vi "pp2_updateSessionInfo.vi"(10 "Session info In":T1, 11 "State In":T2={"Curr  tr"=0, "Curr (ms)"=0, "Cum (ms)"=0, "Run loop diff"=0, "Tone countdown (ms)"=0, "Countdown (ms)"=0, "Curr State"=enum."0 NULL", "Prev State"=enum."0 NULL", "Null"=FALSE, "Sw"=FALSE, "Tone\nGate"=FALSE, "Stim"=FALSE, "Current DAQ DO Int"=0, "Current Loaded Trial"={"Trial Type Number"=1, "Trial Type"=enum."GO", "Trial Weight"=100, "Shock (mA)"=0.3, "Duration (ms)"=0.25, "Sound Type"=enum."04 FM Sweep", "Stim P1"=4000.0, "Stim P2"=0.0, "Stim P3"=0.0, "Stim P4"=2000.0}, "Next Trial (for display purposes)"={"Trial Type Number"=1, "Trial Type"=enum."GO", "Trial Weight"=100, "Shock (mA)"=0.3, "Duration (ms)"=0.25, "Sound Type"=enum."04 FM Sweep", "Stim P1"=4000.0, "Stim P2"=0.0, "Stim P3"=0.0, "Stim P4"=2000.0}, "Total trials memo"=0, "State start cum memo (ms)"=0, "Last dur jump time memo (ms)"=0, "Last dur shock time memo (ms)"=0, "Tone repeat memo (ms)"=0, "Webcam on"=FALSE, "Webcam recording"=FALSE, "State update flag"=FALSE, "Last loaded shock voltage"=0.0} {"Current DAQ DO Int" format="%016b"; "Next Trial (for display purposes)"."Shock (mA)" min=-1.0 max=5.0; "Next Trial (for display purposes)"."Trial Weight" step=1; "Next Trial (for display purposes)"."Duration (ms)" min=0.0 max=1.0; "Next Trial (for display purposes)"."Trial Type Number" min=1 step=1; "Current Loaded Trial"."Shock (mA)" min=-1.0 max=5.0; "Current Loaded Trial"."Trial Weight" step=1; "Current Loaded Trial"."Duration (ms)" min=0.0 max=1.0; "Current Loaded Trial"."Trial Type Number" min=1 step=1}) -> (2 "Session info Out":T1)   [LabVIEW 2013]
uses:
  pp2_CTL_StateInfo.ctl
  pp2_CTL_State.ctl
  pp2_Trial.ctl
  pp2_CTL_TrialType.ctl
  labolabo2/waveforms/WFTypes.ctl
  pp2_CTL_SessionInfo.ctl
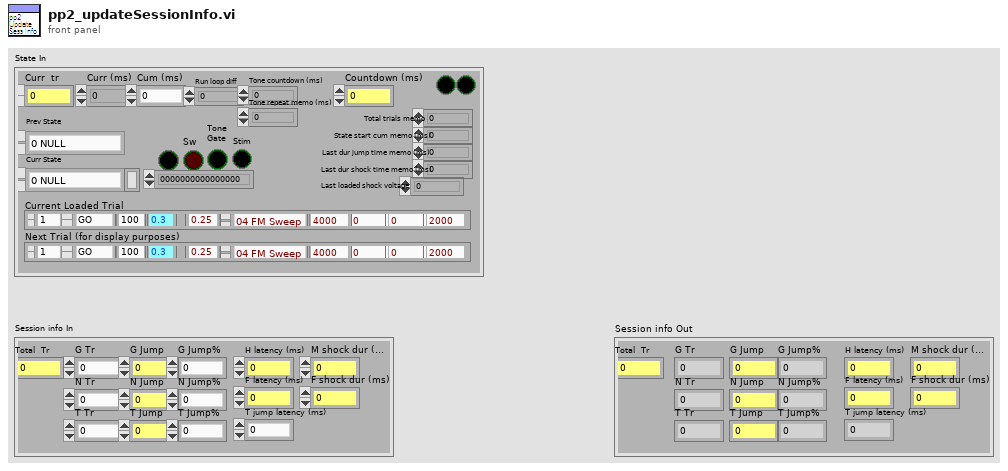
[diagram p1: front panel]
types:
  T1 = typedef "pp2_CTL_SessionInfo.ctl" = cluster{"Total  Tr":u32, "G Tr":u32, "G Jump":u32, "G Jump%":dbl, "N Tr":u32, "N Jump":u32, "N Jump%":dbl, "T Tr":u32, "T Jump":u32, "T Jump%":dbl, "M shock dur (ms)":dbl, "F shock dur (ms)":dbl, "H latency (ms)":dbl, "F latency (ms)":dbl, "T jump latency (ms)":dbl}
  T2 = typedef "pp2_CTL_StateInfo.ctl" = cluster{"Curr  tr":u16, "Curr (ms)":u32, "Cum (ms)":i64, "Run loop diff":i64, "Tone countdown (ms)":i64, "Countdown (ms)":i64, "Curr State":T3, "Prev State":T3, "Null":bool, "Sw":bool, "Tone\nGate":bool, "Stim":bool, "Current DAQ DO Int":u16, "Current Loaded Trial":T4, "Next Trial (for display purposes)":T4, "Total trials memo":i64, "State start cum memo (ms)":i64, "Last dur jump time memo (ms)":i64, "Last dur shock time memo (ms)":i64, "Tone repeat memo (ms)":i64, "Webcam on":bool, "Webcam recording":bool, "State update flag":bool, "Last loaded shock voltage":dbl}
  T3 = typedef "pp2_CTL_State.ctl" = enum8{"0 NULL", "1 Habituation", "2 (Load Trial)", "3 Stay Period", "4 Load Audio/Click Delay", "5 GO Trial", "6 GO Jumped", "7 GO Timeout", "8 NOGO Trial", "9 NOGO Jumped", "10 NOGO Timeout", "11 TEST Trial", "12 TEST Jumped", "13 TEST Timeout", "14 Intertrial Interval", "15 Done"}
  T4 = typedef "pp2_Trial.ctl" = cluster{"Trial Type Number":u8, "Trial Type":T5, "Trial Weight":u32, "Shock (mA)":dbl, "Duration (ms)":dbl, "Sound Type":T6, "Stim P1":dbl, "Stim P2":dbl, "Stim P3":dbl, "Stim P4":dbl}
  T5 = typedef "pp2_CTL_TrialType.ctl" = enum16{"OFF", "GO", "NOGO", "TEST"}
  T6 = typedef "WFTypes.ctl" = enum16{"00 NULL", "01 DC", "02 Noise", "03 Pure Tone", "04 FM Sweep"}
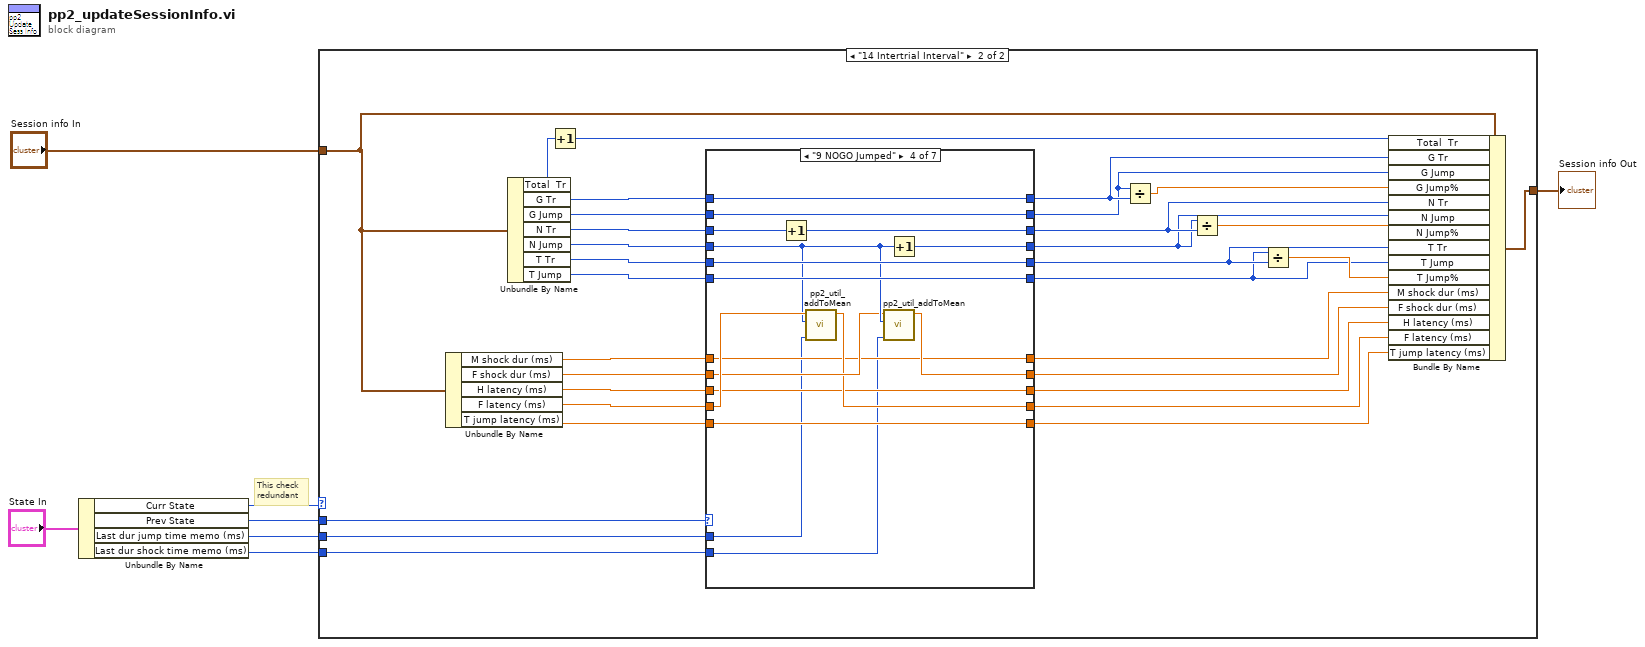
[diagram p0: block diagram]
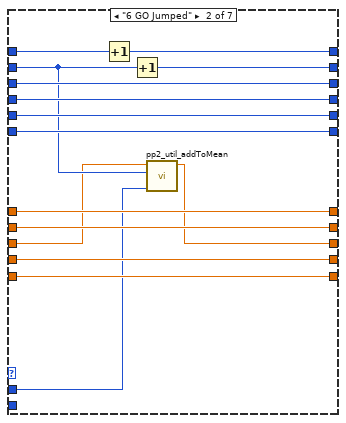
[diagram p4: hidden frame]
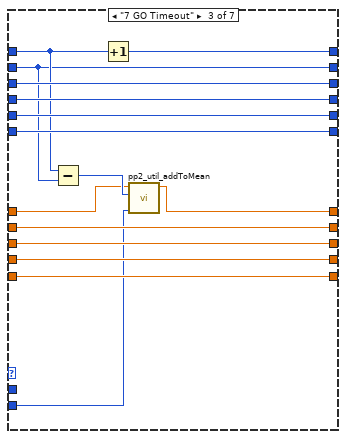
[diagram p5: hidden frame]
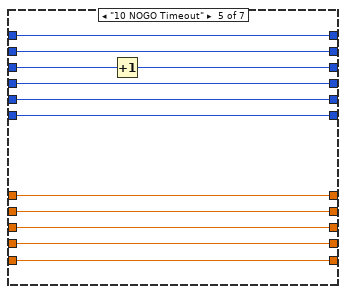
[diagram p6: hidden frame]
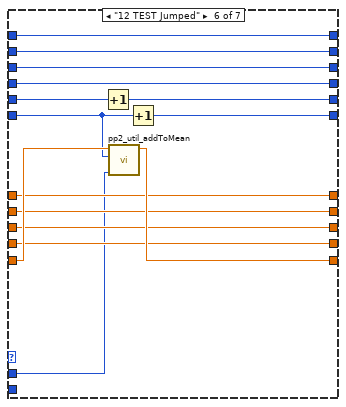
[diagram p7: hidden frame]
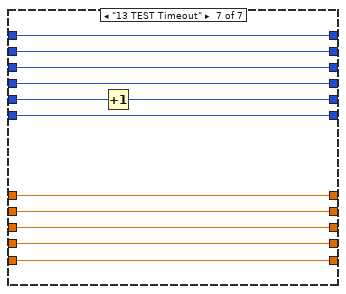
[diagram p8: hidden frame]
diagram:
  # "This check\nredundant"
  n1 = Unbundle By Name("State In") -> ("Curr State"=w1:T3, "Prev State"=w6:T3, "Last dur jump time memo (ms)"=w4:i64, "Last dur shock time memo (ms)"=w3:i64)
  n2 = case shown="\"14 Intertrial Interval\"" w1 {
    tunnel: w6 -> [_ w23]
    tunnel: [w8 w22] -> w5
    tunnel: w4 -> [_ w21]
    tunnel: w3 -> [_ w20]
    tunnel: "Session info In" -> [w8 w14]
    frame Default {
    }
    frame "14 Intertrial Interval" {
      n3 = Unbundle By Name(w14) -> ("M shock dur (ms)"=w13:dbl, "F shock dur (ms)"=w9:dbl, "H latency (ms)"=w10:dbl, "F latency (ms)"=w11:dbl, "T jump latency (ms)"=w12:dbl)
      n4 = Unbundle By Name(w14) -> ("Total  Tr"=w40:u32, "G Tr"=w38:u32, "G Jump"=w37:u32, "N Tr"=w36:u32, "N Jump"=w35:u32, "T Tr"=w34:u32, "T Jump"=w33:u32)
      n5 = Increment(x=w40) -> (x+1=w39:u32)
      n6 = case shown="\"9 NOGO Jumped\"" w23 {
        tunnel: w38 -> [w51 w62 w76 w94 w107 w124 w136]
        tunnel: w37 -> [w50 w55 w75 w95 w108 w125 w137]
        tunnel: w36 -> [w49 w66 w80 w97 w110 w122 w134]
        tunnel: w35 -> [w48 w65 w79 w90 w104 w123 w135]
        tunnel: w34 -> [w47 w64 w78 w93 w106 w121 w133]
        tunnel: w33 -> [w46 w63 w77 w92 w105 w117 w131]
        tunnel: [w49 w66 w80 w96 w109 w122 w134] -> w27
        tunnel: [w48 w65 w79 w98 w104 w123 w135] -> w26
        tunnel: [w47 w64 w78 w93 w106 w120 w132] -> w25
        tunnel: [w46 w63 w77 w92 w105 w119 w131] -> w24
        tunnel: [w51 w61 w81 w94 w107 w124 w136] -> w29
        tunnel: [w50 w56 w75 w95 w108 w125 w137] -> w28
        tunnel: w13 -> [w45 w60 w69 w84 w103 w115 w130]
        tunnel: w9 -> [w44 w59 w71 w89 w102 w114 w129]
        tunnel: w10 -> [w41 w54 w74 w85 w101 w113 w128]
        tunnel: w11 -> [w42 w58 w73 w91 w100 w112 w127]
        tunnel: w12 -> [w43 w57 w72 w86 w99 w118 w126]
        tunnel: w21 -> [_ w52 _ w83 _ w111 _]
        tunnel: w20 -> [_ _ w67 w82 _ _ _]
        tunnel: [w45 w60 w68 w84 w103 w115 w130] -> w19
        tunnel: [w44 w59 w71 w88 w102 w114 w129] -> w18
        tunnel: [w43 w57 w72 w86 w99 w116 w126] -> w15
        tunnel: [w42 w58 w73 w87 w100 w112 w127] -> w16
        tunnel: [w41 w53 w74 w85 w101 w113 w128] -> w17
        frame Default {
        }
        frame "6 GO Jumped" {
          n7 = Increment(x=w62) -> (x+1=w61:u32)
          n8 = Increment(x=w55) -> (x+1=w56:u32)
          n9 = call "pp2_util_addToMean.vi"("New value"=w52, "Original count"=w55, "Original mean"=w54) -> ("New mean"=w53:dbl)  [unwired: 8 in]
        }
        frame "7 GO Timeout" {
          n10 = Subtract(x=w76, y=w75) -> (x-y=w70:u32)
          n11 = Increment(x=w76) -> (x+1=w81:u32)
          n12 = call "pp2_util_addToMean.vi"("New value"=w67, "Original count"=w70, "Original mean"=w69) -> ("New mean"=w68:dbl)  [unwired: 8 in]
        }
        frame "9 NOGO Jumped" {
          n13 = Increment(x=w97) -> (x+1=w96:u32)
          n14 = call "pp2_util_addToMean.vi"("New value"=w83, "Original count"=w90, "Original mean"=w91) -> ("New mean"=w87:dbl)  [unwired: 8 in]
          n15 = call "pp2_util_addToMean.vi"("New value"=w82, "Original count"=w90, "Original mean"=w89) -> ("New mean"=w88:dbl)  [unwired: 8 in]
          n16 = Increment(x=w90) -> (x+1=w98:u32)
        }
        frame "10 NOGO Timeout" {
          n17 = Increment(x=w110) -> (x+1=w109:u32)
        }
        frame "12 TEST Jumped" {
          n18 = Increment(x=w121) -> (x+1=w120:u32)
          n19 = call "pp2_util_addToMean.vi"("New value"=w111, "Original count"=w117, "Original mean"=w118) -> ("New mean"=w116:dbl)  [unwired: 8 in]
          n20 = Increment(x=w117) -> (x+1=w119:u32)
        }
        frame "13 TEST Timeout" {
          n21 = Increment(x=w133) -> (x+1=w132:u32)
        }
      }
      n22 = Divide(x=w28, y=w29) -> (x/y=w32:dbl)
      n23 = Divide(x=w26, y=w27) -> (x/y=w31:dbl)
      n24 = Divide(x=w24, y=w25) -> (x/y=w30:dbl)
      n25 = Bundle By Name(cluster=w14, "Total  Tr"=w39, "G Tr"=w29, "G Jump"=w28, "G Jump%"=w32, "N Tr"=w27, "N Jump"=w26, "N Jump%"=w31, "T Tr"=w25, "T Jump"=w24, "T Jump%"=w30, "M shock dur (ms)"=w19, "F shock dur (ms)"=w18, "H latency (ms)"=w17, "F latency (ms)"=w16, "T jump latency (ms)"=w15) -> (w22:T1)
    }
  }
  "Session info Out" <- w5
